vi "Write Chunk to Stream.vi"(8 "error in (no error)":errorcluster, 10 "Chunk":string, 11 "Stream in":refnum<k5>) -> (0 "error out":errorcluster, 3 "Stream out":refnum<k5>)   [LabVIEW 2020, in "HTTP Utils.lvlib" / "Streamable Response.lvclass"]
uses:
  Streamable Response.lvclass
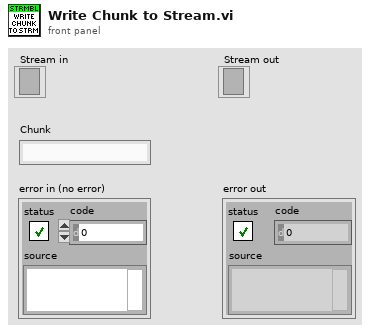
[diagram p1: front panel]
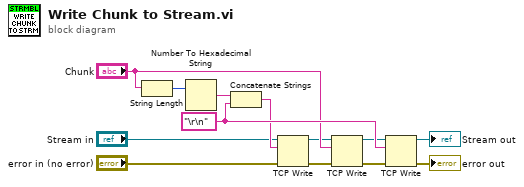
[diagram p0: block diagram]
diagram:
  w6 = "\r\n" ("string")
  n1 = String Length(string="Chunk") -> (length=w13:i32)
  n2 = Number To Hexadecimal String(2:w13) -> (0:w12:string)  [unwired: 1 in]
  n3 = Concatenate Strings(w12, w6) -> (w4:string)
  n4 = TCP Write(connection ID="Stream in", data in=w4, error in (no error)="error in (no error)") -> (connection ID out=w2:refnum<k5>, error out=w8:errorcluster)  [unwired: 1 in, 1 out]
  n5 = TCP Write(connection ID=w2, data in="Chunk", error in (no error)=w8) -> (connection ID out=w1:refnum<k5>, error out=w7:errorcluster)  [unwired: 1 in, 1 out]
  n6 = TCP Write(connection ID=w1, data in=w6, error in (no error)=w7) -> (connection ID out=→"Stream out":refnum<k5>, error out=→"error out":errorcluster)  [unwired: 1 in, 1 out]
